vi "UnitTest-DeleteExistingFilesOrFolders.vi"(8 "error in (no error)":errorcluster, 10 "Config IN":T1={"TableLogger"=enum."CSV Logger", "DB File Path"=path "", "DB Backup Config"={"Directory"=path "", "UTC Time Format"=FALSE, "On Launch"=FALSE, "Interval (Hours)"=-1.0, "Size Multiples (Bytes)"=10000}}) -> (0 "error out":errorcluster)   [LabVIEW 2014]
uses:
  TableLogger_Actor/TableLoggerConfig.ctl
  TableLogger_Actor/TableLoggerTypes.ctl
  TableLogger_Actor/TableLoggerBackupConfig.ctl
  <userlib>/_OpenG.lib/file/file.llb/File Exists - Scalar__ogtk.vi
  TableLogger_Actor/TableLogger_Actor.lvlib
panel:
  # "Connector Pane"
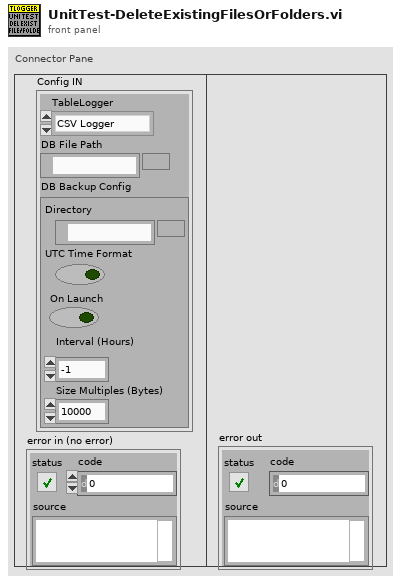
[diagram p1: front panel]
types:
  T1 = typedef "TableLogger_Actor.lvlib/TableLoggerConfig.ctl" = cluster{"TableLogger":T2, "DB File Path":path, "DB Backup Config":T3}
  T2 = typedef "TableLogger_Actor.lvlib/TableLoggerTypes.ctl" = enum16{"CSV Logger", "SQLite Logger"}
  T3 = typedef "TableLogger_Actor.lvlib/TableLoggerBackupConfig.ctl" = cluster{"Directory":path, "UTC Time Format":bool, "On Launch":bool, "Interval (Hours)":dbl, "Size Multiples (Bytes)":i32}
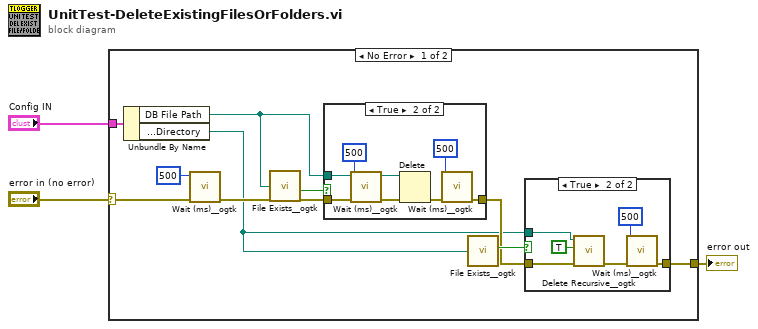
[diagram p0: block diagram]
diagram:
  n1 = case shown="No Error" "error in (no error)" {
    selector: "error in (no error)" -> [w11 w29]
    tunnel: [w9 w29] -> w2
    tunnel: "Config IN" -> [w6 _]
    frame No Error {
      n2 = Unbundle By Name(w6) -> ("DB File Path"=w5:path, "DB Backup Config.Directory"=w4:path)
      n3 = call <userlib>:"Wait (ms)__ogtk.vi"("error in (no error)"=w11, "milliseconds to wait"=u32 500) -> ("error out"=w8:errorcluster)  [unwired: 8 in, 1 out]
      n4 = call-poly <userlib>:"File Exists__ogtk.vi"("file path"=w5) -> ("exists"=w13:bool)  [unwired: 6 in, 1 out]
      n5 = case shown="True" w13 {
        tunnel: [w14 w20] -> w10
        tunnel: w5 -> [_ w18]
        tunnel: w8 -> [w14 w16]
        frame False {
        }
        frame True {
          n6 = call <userlib>:"Wait (ms)__ogtk.vi"("error in (no error)"=w16, "milliseconds to wait"=u32 500) -> ("error out"=w15:errorcluster)  [unwired: 8 in, 1 out]
          n7 = Delete(path (use dialog)=w18, error in=w15) -> (error out=w21:errorcluster)  [unwired: 3 in, 2 out]
          n8 = call <userlib>:"Wait (ms)__ogtk.vi"("error in (no error)"=w21, "milliseconds to wait"=u32 500) -> ("error out"=w20:errorcluster)  [unwired: 8 in, 1 out]
        }
      }
      n9 = call-poly <userlib>:"File Exists__ogtk.vi"("file path"=w4) -> ("is directory"=w12:bool)  [unwired: 6 in, 1 out]
      n10 = case shown="True" w12 {
        tunnel: w4 -> [_ w27]
        tunnel: [w22 w23] -> w9
        tunnel: w10 -> [w22 w26]
        frame False {
        }
        frame True {
          n11 = call <userlib>:"Delete Recursive__ogtk.vi"("error in (no error)"=w26, "Recursive? (FALSE)"=TRUE, "Path"=w27) -> ("error out"=w24:errorcluster)  [unwired: 7 in, 1 out]
          n12 = call <userlib>:"Wait (ms)__ogtk.vi"("error in (no error)"=w24, "milliseconds to wait"=u32 500) -> ("error out"=w23:errorcluster)  [unwired: 8 in, 1 out]
        }
      }
    }
    frame Error {
    }
  }
  "error out" <- w2
